vi "Header_CF.vi"(1 "Cluster":T1={"Multiply Data?"=TRUE, "Configuration"=enum."Preamp", "Preamp Sensitivity"=enum."1nA/V", "Step Time (sec)"=0.5, "Output 1"=0.0, "Output 2"=0.0, "Preamp Bias (mv)"=0, "Preamp Bias on?"=FALSE, "Wavelength:"=1010.0, "Use Current offset"=TRUE, "Current offset"=0.0, "Y scale 1"="", "x scale"="", "Vis path"=path "", "IR path"=path ""} {"Wavelength:" min=0.0 max=2000.0 step=0.1 format="%.1f"; "Output 2" step=0.05; "Output 1" step=0.01; "Step Time (sec)" min=0.001 max=300.0 step=0.001 format="%.3f"}, 2 "String in":string) -> (0 "String out":string)   [LabVIEW 2013]
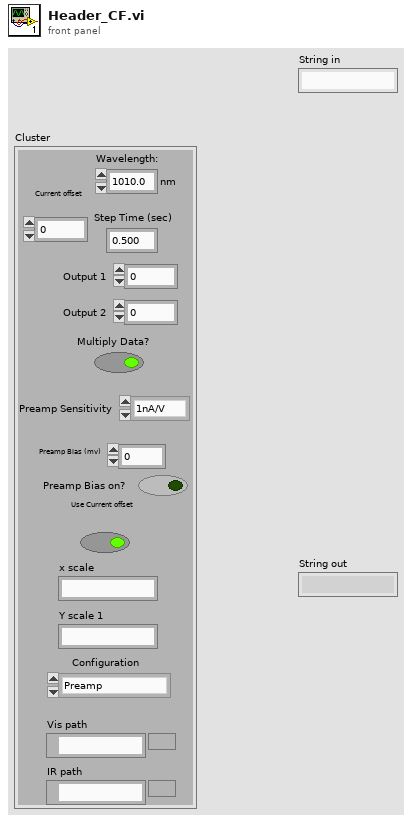
[diagram p1: front panel]
types:
  T1 = cluster{"Multiply Data?":bool, "Configuration":enum16{"Preamp to Lockin", "Preamp", "Lockin current", "Lockin Voltage", ""}, "Preamp Sensitivity":enum16{"1pA/V", "2pA/V", "5pA/V", "10pA/V", "20pA/V", "50pA/V", "100pA/V", "200pA/V", "500pA/V", "1nA/V", "2nA/V", "5nA/V", "10nA/V", "20nA/V", "50nA/V", "100nA/V", "200nA/V", "500nA/V", "1uA/V", "2uA/V", "5uA/V", "10uA/V", "20uA/V", "50uA/V", "100uA/V", "200uA/V", "500uA/V", "1mA/V"}, "Step Time (sec)":dbl, "Output 1":dbl, "Output 2":dbl, "Preamp Bias (mv)":i32, "Preamp Bias on?":bool, "Wavelength:":dbl, "Use Current offset":bool, "Current offset":dbl, "Y scale 1":string, "x scale":string, "Vis path":path, "IR path":path}
  T2 = enum16{"Preamp to Lockin", "Preamp", "Lockin current", "Lockin Voltage", ""}
  T3 = enum16{"1pA/V", "2pA/V", "5pA/V", "10pA/V", "20pA/V", "50pA/V", "100pA/V", "200pA/V", "500pA/V", "1nA/V", "2nA/V", "5nA/V", "10nA/V", "20nA/V", "50nA/V", "100nA/V", "200nA/V", "500nA/V", "1uA/V", "2uA/V", "5uA/V", "10uA/V", "20uA/V", "50uA/V", "100uA/V", "200uA/V", "500uA/V", "1mA/V"}
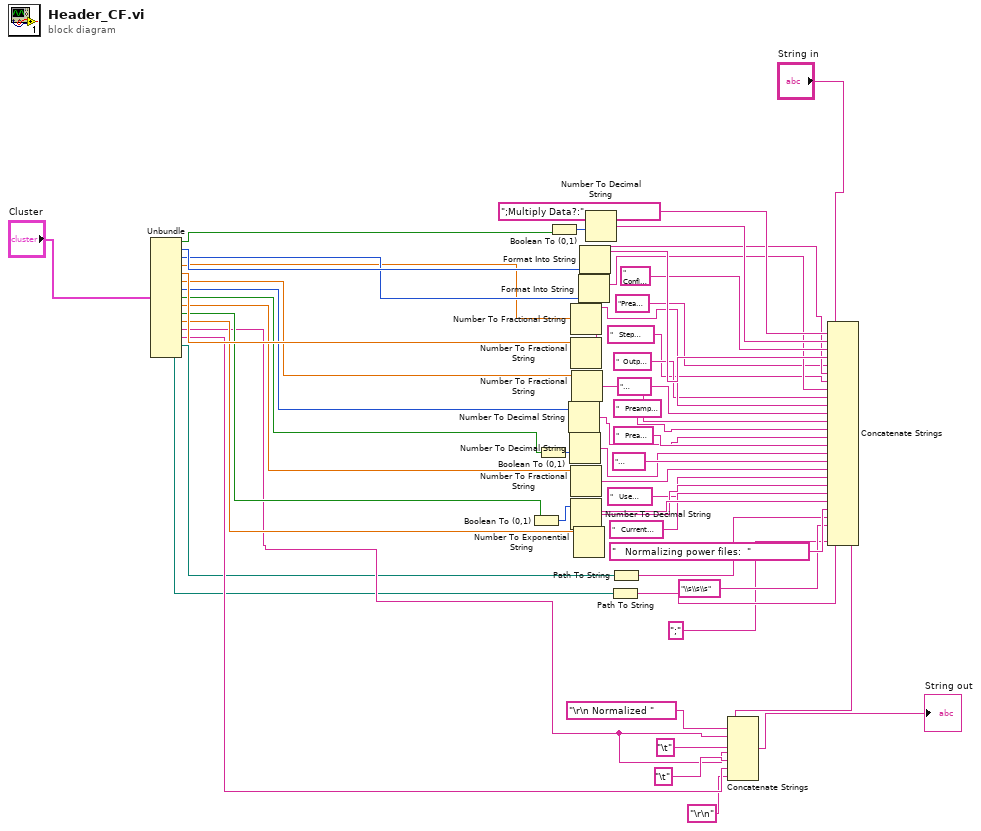
[diagram p0: block diagram]
diagram:
  n1 = Unbundle("Cluster") -> ("Multiply Data?"=w21:bool, "Configuration"=w20:T2, "Preamp Sensitivity"=w19:T3, "Step Time (sec)"=w18:dbl, "Output 1"=w17:dbl, "Output 2"=w16:dbl, "Preamp Bias (mv)"=w15:i32, "Preamp Bias on?"=w14:bool, "Wavelength:"=w13:dbl, "Use Current offset"=w12:bool, "Current offset"=w11:dbl, "Y scale 1"=w10:string, "x scale"=w9:string, "Vis path"=w8:path, "IR path"=w7:path)
  n2 = Boolean To (0,1)(Boolean=w12) -> (0, 1=w49:i16)
  n3 = Boolean To (0,1)(Boolean=w14) -> (0, 1=w25:i16)
  n4 = Boolean To (0,1)(Boolean=w21) -> (0, 1=w40:i16)
  n5 = Number To Decimal String(number=w15) -> (decimal integer string=w33:string)  [unwired: 1 in]
  n6 = Number To Decimal String(number=w25) -> (decimal integer string=w35:string)  [unwired: 1 in]
  n7 = Number To Fractional String(number=w18) -> (F-format string=w28:string)  [unwired: 3 in]
  n8 = Number To Fractional String(number=w17) -> (F-format string=w30:string)  [unwired: 3 in]
  n9 = Number To Fractional String(number=w13) -> (F-format string=w43:string)  [unwired: 3 in]
  n10 = Number To Decimal String(number=w49) -> (decimal integer string=w51:string)  [unwired: 1 in]
  n11 = Number To Fractional String(number=w16) -> (F-format string=w48:string)  [unwired: 3 in]
  n12 = Number To Exponential String(number=w11) -> (E-format string=w53:string)  [unwired: 3 in]
  n13 = Format Into String(w19) -> (resulting string=w36:string)  [unwired: 3 in, 1 out]
  n14 = Format Into String(w20) -> (resulting string=w38:string)  [unwired: 3 in, 1 out]
  n15 = Number To Decimal String(number=w40) -> (decimal integer string=w41:string)  [unwired: 1 in]
  n16 = Path To String(path=w7) -> (string=w3:string)
  n17 = Path To String(path=w8) -> (string=w5:string)
  n18 = Concatenate Strings("String in", ";Multiply Data?:" ("string"), w41, "  Configuration:" ("string"), w38, "Preamp Sensitivity:" ("string"), w36, "   Step Time:" ("string"), w28, "  Output 1 :" ("string"), w30, "   Output 2:" ("string"), w48, "   Preamp Bias:" ("string"), w33, "   Preamp Bias on: " ("string"), w35, "   Wavelength: " ("string"), w43, "   Use Current offset: " ("string"), w51, "   Current offset: " ("string"), w53, "   Normalizing power files:  ", w5, "\\s\\s\\s", w3, ";" ("string")) -> (w44:string)
  n19 = Concatenate Strings(w44, "\r\n Normalized " ("string"), w10, "\t" ("string"), w10, "\t" ("string"), w9, "\r\n" ("string")) -> (→"String out":string)
